vi "Pre-bias Cell.vi"(9 "Scan Settings JV":T1={"Light intensity (Suns)"=1.0, "Pre-bias time (s)"=5.0, "Maximum voltage (V)"=0.0, "Minimum voltage (V)"=-1.4, "Range Options"=0, "1st scan FB to SC?"=TRUE, "Step Size (V)"=0.01, "Source Delay (s)"=0.01, "Inverted device"=FALSE, "Measure stabilized power output"=TRUE, "Stabilzation time (s)"=40.0, "Use Vmp from JV scan"=TRUE, "Stabization voltage (V)"=0.8, "Only stabilize best pixels"=TRUE, "Number of pixels to stabilize \nper substrate"=0, "Stabilization time step (s)"=1.0, "Use max power tracking"=FALSE, "Pre-bias voltage (V)"=-1.4, "No. of data point averages"=1.0, "No. of J-V averages"=1.0, "Integration time (ms)"=200.0} {"Number of pixels to stabilize \nper substrate" items=["1", "2", "3", "4", "5", "6", "7", "8"]; "Range Options" items=["Auto Range", "Semi-Auto Range", "100 uA", "1 mA", "10 mA", "100 mA", "1A"]}, 11 "VISA resource name":refnum<visa-resource-name>="GPIB0::24::INSTR") -> (0 "error out":errorcluster, 3 "VISA resource name out":refnum<visa-resource-name>)   [LabVIEW 2011]
uses:
  Typedefs/Scan settings.ctl
  <instrlib>/Keithley 24XX/Public/Data/Read (Single Point).vi
  <instrlib>/Keithley 24XX/Keithley 24XX.lvlib
panel:
  in  "Manual Range (1.0)":dbl=1.0
  in  "Source Mode  (0: Voltage)":u16(ring) items=["Voltage", "Current"]
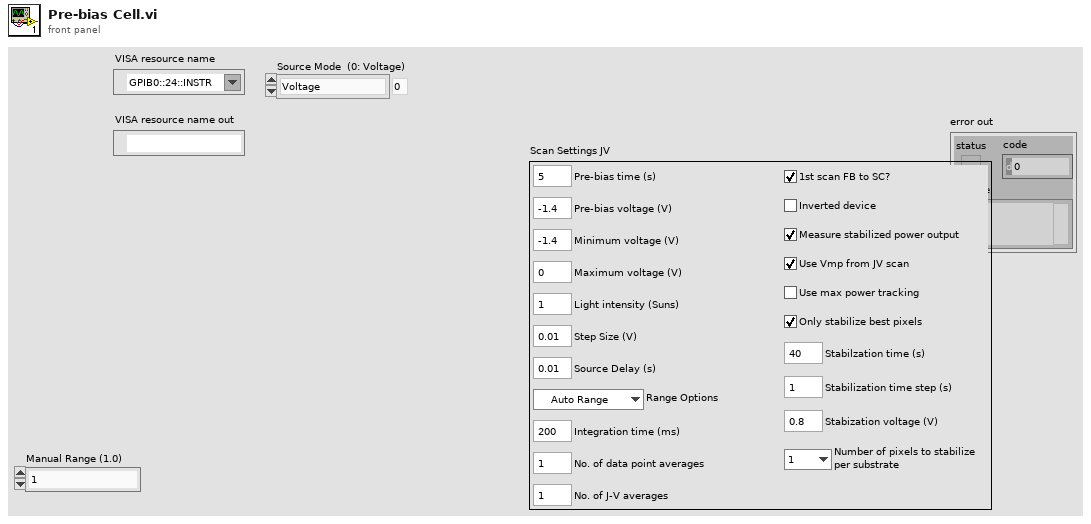
[diagram p1: front panel]
types:
  T1 = typedef "Scan settings.ctl" = cluster{"Light intensity (Suns)":dbl, "Pre-bias time (s)":dbl, "Maximum voltage (V)":dbl, "Minimum voltage (V)":dbl, "Range Options":u16, "1st scan FB to SC?":bool, "Step Size (V)":dbl, "Source Delay (s)":dbl, "Inverted device":bool, "Measure stabilized power output":bool, "Stabilzation time (s)":dbl, "Use Vmp from JV scan":bool, "Stabization voltage (V)":dbl, "Only stabilize best pixels":bool, "Number of pixels to stabilize \nper substrate":u16, "Stabilization time step (s)":dbl, "Use max power tracking":bool, "Pre-bias voltage (V)":dbl, "No. of data point averages":dbl, "No. of J-V averages":dbl, "Integration time (ms)":dbl}
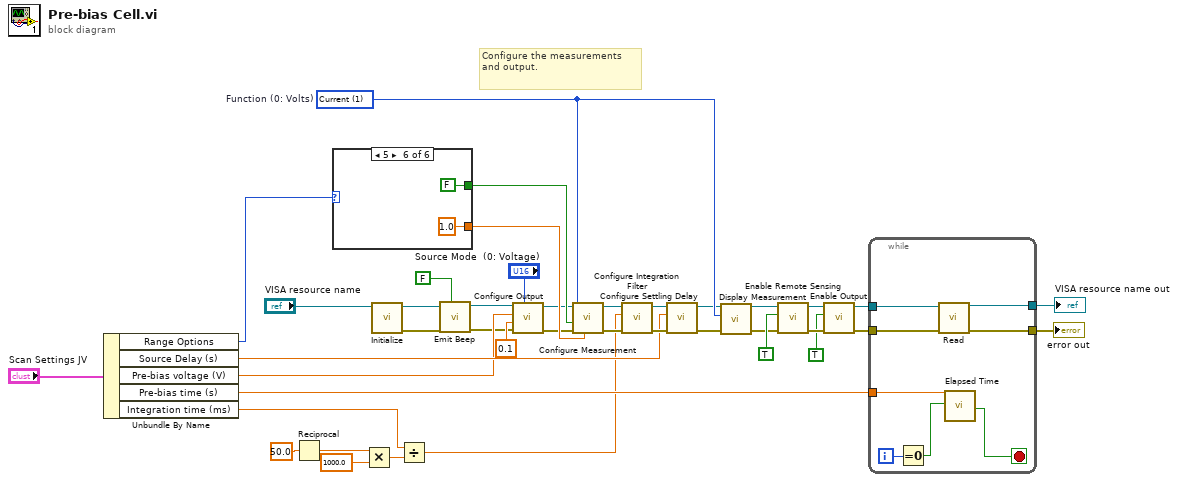
[diagram p0: block diagram]
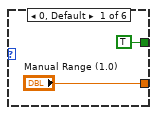
[diagram p2: hidden frame]
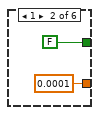
[diagram p3: hidden frame]
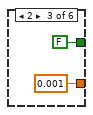
[diagram p4: hidden frame]
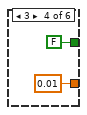
[diagram p5: hidden frame]
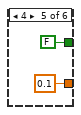
[diagram p6: hidden frame]
diagram:
  w26 = u16 1 items=["Volts", "Current", "Resistance"]  # Function (0: Volts)
  # "Configure the measurements and output."
  n1 = Unbundle By Name("Scan Settings JV") -> ("Range Options"=w7:u16, "Source Delay (s)"=w18:dbl, "Pre-bias voltage (V)"=w17:dbl, "Pre-bias time (s)"=w16:dbl, "Integration time (ms)"=w2:dbl)
  n2 = Reciprocal(x=50.0) -> (1/x=w4:dbl)
  n3 = case shown="5" w7 {
    tunnel: ["Manual Range (1.0)" 0.0001 ("Manual Range (1.0)") 0.001 ("Manual Range (1.0)") 0.01 ("Manual Range (1.0)") 0.1 ("Manual Range (1.0)") 1.0 ("Manual Range (1.0)")] -> w14
    tunnel: [TRUE FALSE FALSE FALSE FALSE FALSE] -> w15
    frame 0, Default {
    }
    frame 1 {
    }
    frame 2 {
    }
    frame 3 {
    }
    frame 4 {
    }
    frame 5 {
    }
  }
  n4 = Multiply(x=w4, y=1000.0) -> (x*y=w3:dbl)
  n5 = call <instrlib>:"Initialize.vi"("VISA resource name"="VISA resource name") -> ("error out"=w23:errorcluster, "VISA resource name out"=w24:refnum<visa-resource-name>)  [unwired: 9 in]
  n6 = Divide(x=w2, y=w3) -> (x/y=w1:dbl)
  n7 = call <instrlib>:"Emit Beep.vi"("Enable Beep (F)"=FALSE, "error in (no error)"=w23, "VISA resource name"=w24) -> ("error out"=w12:errorcluster, "VISA resource name out"=w13:refnum<visa-resource-name>)  [unwired: 7 in]
  n8 = call <instrlib>:"Configure Output.vi"("Source Mode  (0: Voltage)"="Source Mode  (0: Voltage)", "error in (no error)"=w12, "Compliance  Level (0.1)"=0.1, "Output Level (0)"=w17, "VISA resource name"=w13) -> ("error out"=w10:errorcluster, "VISA resource name out"=w11:refnum<visa-resource-name>)  [unwired: 5 in]
  n9 = call <instrlib>:"Configure Measurement.vi"("Manual Range (1.0)"=w14, "error in (no error)"=w10, "Enable Auto Range (T:Enable)"=w15, "Function (0: Volts)"=w26, "VISA resource name"=w11) -> ("error out"=w29:errorcluster, "VISA resource name out"=w30:refnum<visa-resource-name>)  [unwired: 5 in]
  n10 = call <instrlib>:"Configure Integration Filter.vi"("error in (no error)"=w29, "Measurement Speed (1 PLC)"=w1, "VISA resource name"=w30) -> ("error out"=w20:errorcluster, "VISA resource name out"=w21:refnum<visa-resource-name>)  [unwired: 7 in]
  n11 = call <instrlib>:"Configure Settling Delay.vi"("error in (no error)"=w20, "Manual Settling Delay (0 sec)"=w18, "VISA resource name"=w21) -> ("error out"=w8:errorcluster, "VISA resource name out"=w9:refnum<visa-resource-name>)  [unwired: 7 in]
  n12 = call <instrlib>:"Display Measurement.vi"("error in (no error)"=w8, "Displayed Measurement (0: Voltage)"=w26, "VISA resource name"=w9) -> ("error out"=w27:errorcluster, "VISA resource name out"=w28:refnum<visa-resource-name>)  [unwired: 7 in]
  n13 = call <instrlib>:"Enable Remote Sensing.vi"("error in (no error)"=w27, "Enable Remote Sensing (T: Enable)"=TRUE ("Enable Output (T: Enable)"), "VISA resource name"=w28) -> ("error out"=w33:errorcluster, "VISA resource name out"=w34:refnum<visa-resource-name>)  [unwired: 7 in]
  n14 = call <instrlib>:"Enable Output.vi"("error in (no error)"=w33, "Enable Output (T: Enable)"=TRUE, "VISA resource name"=w34) -> ("error out"=w39:errorcluster, "VISA resource name out"=w38:refnum<visa-resource-name>)  [unwired: 7 in]
  n15 = while {
    tunnel: w39 -> [w60]
    tunnel: w38 -> [w59]
    tunnel: [w58] -> w36
    tunnel: [w57] -> w35
    tunnel: w16 -> [w53]
    i -> [w56]
    stop <- w55 stop-if-true
    n16 = Equal To 0?(x=w56) -> (x = 0?=w54:bool)
    n17 = call-poly <instrlib>:"Read.vi"("VISA resource name"=w59, "error in (no error)"=w60) -> ("VISA resource name out"=w57:refnum<visa-resource-name>, "error out"=w58:errorcluster)  [unwired: 7 in, 5 out]
    n18 = call "Elapsed Time"("Time Target (s)"=w53, "Reset"=w54) -> ("Time has Elapsed"=w55:bool)  [unwired: 10 in, 7 out]
  }
  "VISA resource name out" <- w35
  "error out" <- w36
